vi "Exit Loop on Stop or Error.vi"(8 "error in (no error)":errorcluster) -> (0 "error out":errorcluster, 3 "Exit?":bool)   [LabVIEW 2015]
doc: "Exit a loop based on two conditions:\n\n1. An error is detected - Produce a dialog giving the user the option to clear the error and continue or exit the program.\n\n2. A stop command has been issued by another loop in the application."
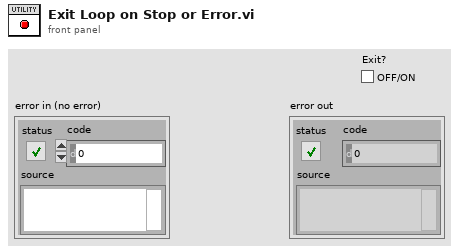
[diagram p1: front panel]
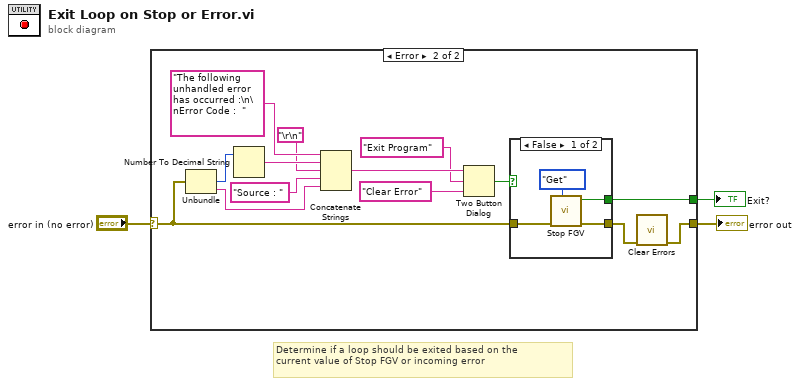
[diagram p0: block diagram]
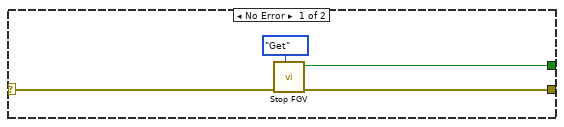
[diagram p2: hidden frame]
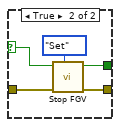
[diagram p3: hidden frame]
diagram:
  # "Determine if a loop should be exited based on the\ncurrent value of Stop FGV or incoming error"
  n1 = case shown="Error" "error in (no error)" {
    selector: "error in (no error)" -> [w6 w19]
    tunnel: [w5 w8] -> w2
    tunnel: [w4 w21] -> w1
    frame No Error {
      n2 = call "Stop FGV.vi"("Mode"=enum16{"Set", "Get"}."Get", "error in (no error)"=w6) -> ("error out (no error)"=w5:errorcluster, "Get Stop Condition"=w4:bool)  [unwired: 8 in]
    }
    frame Error {
      n3 = Unbundle(w19) -> ("code"=w18:i32, "source"=w14:string)  [unwired: 1 out]
      n4 = Number To Decimal String(number=w18) -> (decimal integer string=w17:string)  [unwired: 1 in]
      n5 = Concatenate Strings("The following unhandled error has occurred :\n\nError Code :  ", w17, "\r\n", "Source : ", w14) -> (w13:string)
      n6 = Two Button Dialog(message=w13, 1:"Clear Error", 2:"Exit Program") -> (T button?=w10:bool)
      n7 = case shown="False" w10 {
        selector: w10 -> [_ w26]
        tunnel: [w25 w29] -> w9
        tunnel: [w23 w28] -> w21
        tunnel: w19 -> [w22 w27]
        frame False {
          n8 = call "Stop FGV.vi"("Mode"=enum16{"Set", "Get"}."Get", "error in (no error)"=w22) -> ("error out (no error)"=w25:errorcluster, "Get Stop Condition"=w23:bool)  [unwired: 8 in]
        }
        frame True {
          n9 = call "Stop FGV.vi"("Mode"=enum16{"Set", "Get"}."Set", "error in (no error)"=w27, "Set Stop Condition"=w26) -> ("error out (no error)"=w29:errorcluster, "Get Stop Condition"=w28:bool)  [unwired: 7 in]
        }
      }
      n10 = call <vilib>:"Clear Errors.vi"("error in (no error)"=w9) -> ("error out"=w8:errorcluster)  [unwired: 5 in, 1 out]
    }
  }
  "error out" <- w2
  "Exit?" <- w1
